vi "Go Home.vi"(8 "Side":T1=enum."right") -> ()   [LabVIEW 2013]
uses:
  ROS/Code/SubVIs/BaxterSide.ctl
panel:
  in  "L:Home":dbl[](array[numeric])=[45.0, -45.0, 0.0, 45.0, 0.0, 90.0, 0.0]
  in  "R:Home":dbl[](array[numeric])=[-45.0, -45.0, 0.0, 45.0, 0.0, 90.0, 0.0]
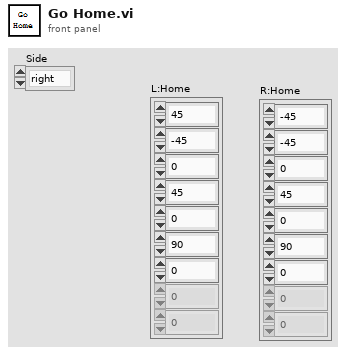
[diagram p1: front panel]
types:
  T1 = typedef "BaxterSide.ctl" = enum16{"left", "right"}
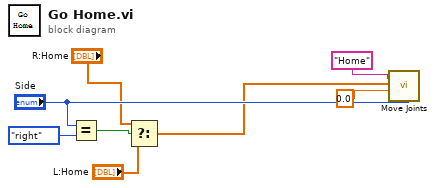
[diagram p0: block diagram]
diagram:
  n1 = Equal?(x="Side", y=BaxterSide."right") -> (x = y?=w4:bool)
  n2 = Select(t="R:Home", s=w4, f="L:Home") -> (s? t:f=w1:dbl[])
  n3 = call "Move Joints.vi"("Side"="Side", "Label"="Home", "time"=0.0, "Goal"=w1) -> ()  [unwired: 6 in, 2 out]
